vi "RunAnimation.vi"() -> ()   [LabVIEW 2018]
panel:
  out "Horizontal Fill Indicator":dbl(slide) scale=0.0..100.0
  # "Tu Credito Pyme BBVA"
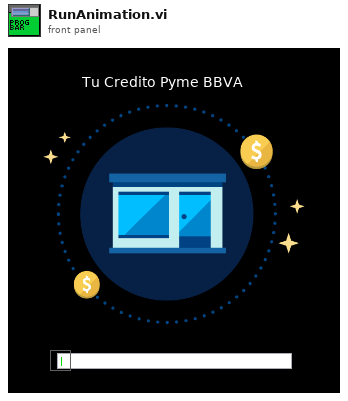
[diagram p1: front panel]
types:
  T1 = enum32{"Invalid", "Standard", "Closed", "Hidden", "Minimized", "Maximized"}
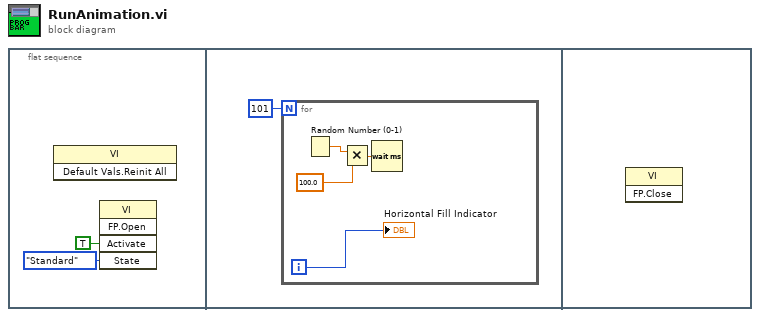
[diagram p0: block diagram]
diagram:
  n1 = flat-sequence {
    frame #0 {
      n2 = invoke class="VI" method="Default Vals.Reinit All"() -> ()  [unwired: 3 in, 3 out]
      n3 = invoke class="VI" method="FP.Open"("Activate"=TRUE ("Activate?"), "State"=T1."Standard") -> ()  [unwired: 3 in, 5 out]
    }
    frame #1 {
      n4 = for {
        N: 101 -> [_]
        i -> [w7]
        n5 = Random Number (0-1)() -> (number: 0 to 1=w6:dbl)
        n6 = Multiply(x=w6, y=100.0) -> (x*y=w4:dbl)
        n7 = Wait (ms)(milliseconds to wait=w4) -> ()  [unwired: 1 out]
        "Horizontal Fill Indicator" <- w7
      }
    }
    frame #2 {
      n8 = invoke class="VI" method="FP.Close"() -> ()  [unwired: 3 in, 3 out]
    }
  }
